vi "CreateTopicActorDescriptor.vi"(8 "error in (no error)":errorcluster, 9 "1:M":bool, 10 "Transport":refnum<class "Message Transport Queue.lvclass">, 11 "Name":string) -> (0 "error out":errorcluster, 3 "Topic Actor Descriptor out":refnum<class "Topic Actor Descriptor.lvclass">)   [LabVIEW 2016, in "Stream Mediator.lvlib" / "Topic Actor Descriptor.lvclass"]
doc: "--\nCopyright © 2017 Composed SystemsI All rights reserved.\n\nAuthor: Jon McBee <jon.mcbee@composed.io>\n\nThis library is provided \"AS IS\" ,WITHOUT WARRANTIES OR\nCONDITIONS OF ANY KIND, either express or implied.\n\nComposed Systems -- composed.io\n\nStream 0.0.1.1\nJon McBee - Composed Systems\nCopyright (c) 2017, Composed Systems"
uses:
  <userlib>/Composed Systems/Stream/Mediator/Classes/Topic Actor Descriptor/Topic Actor Descriptor.lvclass
  <userlib>/Composed Systems/Stream/Mediator/Classes/Message Transport Queue/Message Transport Queue.lvclass
  C:/Program Files (x86)/National Instruments/LabVIEW 2016/user.lib/Composed Systems/Stream/Mediator/Classes/Message Transport Interface/Message Transport Interface.lvclass
  <userlib>/Composed Systems/Stream/Mediator/Classes/Topic Actor Descriptor/Topic Actor Descriptor.lvclass/Topic Actor Descriptor.ctl
  <userlib>/Composed Systems/Stream/Mediator/Classes/Message Transport Interface/Message Transport Interface.lvclass
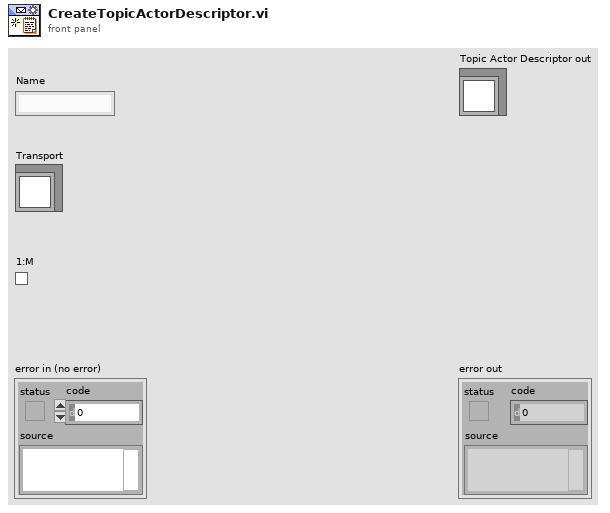
[diagram p1: front panel]
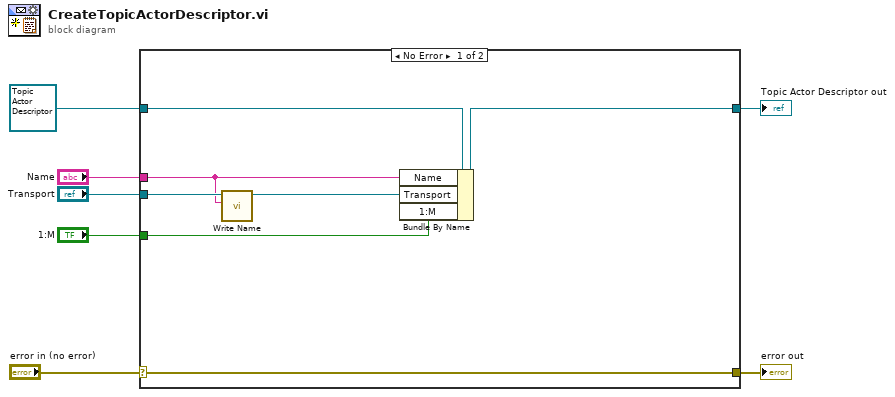
[diagram p0: block diagram]
diagram:
  n1 = case shown="No Error" "error in (no error)" {
    selector: "error in (no error)" -> [w14 w16]
    tunnel: [w14 w16] -> w6
    tunnel: [w11 w15] -> w4
    tunnel: refnum<class "Topic Actor Descriptor.lvclass"> refnum ("Topic Actor Descriptor in") -> [w12 w15]
    tunnel: "Name" -> [w8 _]
    tunnel: "Transport" -> [w10 _]
    tunnel: "1:M" -> [w13 _]
    frame No Error {
      n2 = call <userlib>:"Write Name.vi"("Name"=w8, "Message Transport Interface in"=w10) -> ("Message Transport Interface out"=w9:refnum<class "Message Transport Queue.lvclass">)  [unwired: 8 in, 1 out]
      n3 = Bundle By Name(cluster=w12, "Name"=w8, "Transport"=w9, "1:M"=w13) -> (w11:refnum<class "Topic Actor Descriptor.lvclass">)
    }
    frame Error {
    }
  }
  "error out" <- w6
  "Topic Actor Descriptor out" <- w4
